vi "OP150ZP_SEALING.vi"(8 "ERRIN":errorcluster caption="entrée d'erreur (pas d'erreur)") -> (0 "ERROUT":errorcluster caption="sortie d'erreur", 2 "SEALING_VALUE":dbl, 3 "IsOK?":bool)   [LabVIEW 2020]
uses:
  <instrlib>/HIOKI BT356X Series/HIOKI BT356X Series.lvlib
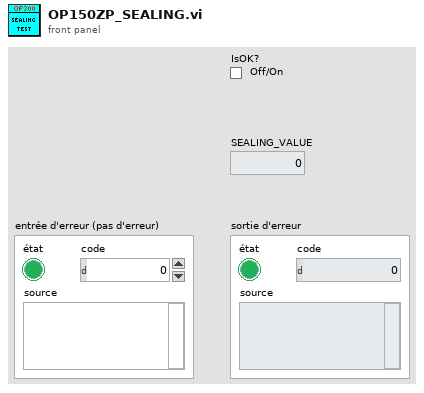
[diagram p1: front panel]
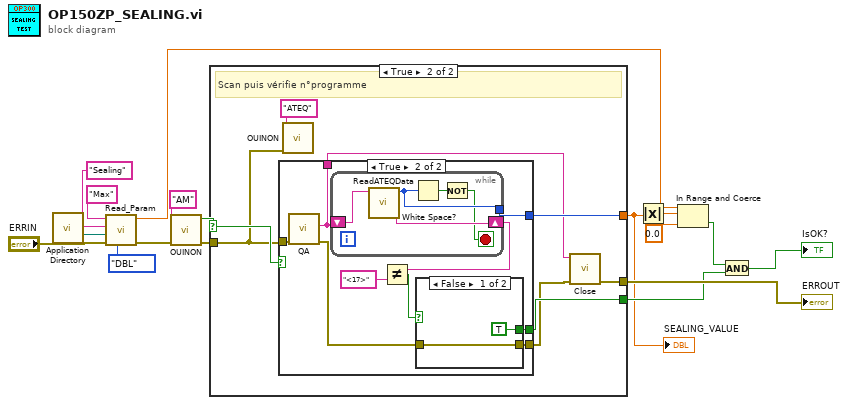
[diagram p0: block diagram]
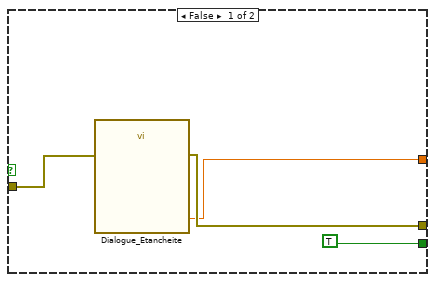
[diagram p2: hidden frame]
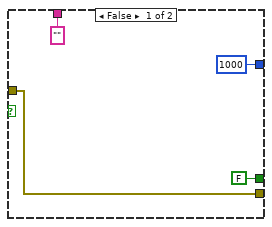
[diagram p3: hidden frame]
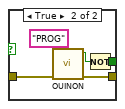
[diagram p4: hidden frame]
diagram:
  n1 = call <vilib>:"Application Directory.vi"() -> ("Application Directory"=w15:path)
  n2 = call "Read_Param.vi"("Énum"=enum16{"STR", "DBL", "U32"}."DBL", "errin"="ERRIN", "pathin"=w15, "section"="Sealing", "key"="Max") -> ("error out"=w6:errorcluster, "dbl"=w10:dbl)  [unwired: 2 in, 3 out]
  n3 = call "OUINON.vi"("errin"=w6, "image"="AM" ("IN")) -> ("error out"=w4:errorcluster, "OUI/NON"=w5:bool)  [unwired: 8 in]
  n4 = case shown="True" w5 {
    selector: w5 -> [_ w26]
    tunnel: [w20 w29] -> w2
    tunnel: [w21 w23] -> w16
    tunnel: [TRUE w28] -> w8
    tunnel: w4 -> [w18 w25]
    frame False {
      n5 = call "Dialogue_Etancheite.vi"("error in (no error)"=w18) -> ("Valeur d'étanchéité"=w20:dbl, "error out"=w21:errorcluster)  [unwired: 16 in, 1 out]
    }
    frame True {
      # "Scan puis vérifie n°programme"
      n6 = case shown="True" w26 {
        tunnel: [1000 ("Valeur") w42] -> w29
        tunnel: [w33 w40] -> w24
        tunnel: [FALSE w39] -> w28
        tunnel: w25 -> [w33 w35]
        tunnel: ["" ("DATAOUT") w34] -> w22
        frame False {
        }
        frame True {
          n7 = call "QA.vi"("ERRIN"=w35) -> ("ERROUT"=w41:errorcluster, "DATAOUT"=w34:string)  [unwired: 9 in]
          n8 = while {
            tunnel: [w47] -> w42
            shift-right: [w45] -> w38
            shift-left: w34 -> [w46]
            stop <- w43 stop-if-true
            n9 = call "ReadATEQData.vi"("Chaîne"=w46) -> ("Prg number"=w45:string, "Valeur"=w47:i32)  [unwired: 7 in, 2 out]
            n10 = White Space?(1:w47) -> (0:w44:bool)
            n11 = Not(x=w44) -> (.not. x?=w43:bool)
          }
          n12 = Not Equal?(x=w38, y="<17>") -> (x != y?=w36:bool)
          n13 = case shown="False" w36 {
            tunnel: w41 -> [w48 w53]
            tunnel: [w48 w52] -> w40
            tunnel: [TRUE w50] -> w39
            frame False {
            }
            frame True {
              n14 = call "OUINON.vi"("errin"=w53, "image"="PROG" ("IN")) -> ("error out"=w52:errorcluster, "OUI/NON"=w51:bool)  [unwired: 8 in]
              n15 = Not(x=w51) -> (.not. x?=w50:bool)
            }
          }
        }
      }
      n16 = call "OUINON.vi"("errin"=w25, "image"="ATEQ" ("IN")) -> ()  [unwired: 8 in, 2 out]
      n17 = call <instrlib>:"Close.vi"("error in (no error)"=w24, "VISA resource name"=w22) -> ("error out"=w23:errorcluster)  [unwired: 9 in]
    }
  }
  "SEALING_VALUE" <- w2
  "ERROUT" <- w16
  n18 = Absolute Value(x=w2) -> (abs(x)=w1:dbl)
  n19 = In Range and Coerce ("Dans la gamme")(upper limit=w10, x=w1, lower limit=0.0 ("limite inférieure")) -> (In Range?=w9:bool)  [unwired: 1 out]
  n20 = And(x=w9, y=w8) -> (x .and. y?=→"IsOK?":bool)
